vi "Angle.vi"() -> ()   [LabVIEW 2012]
panel:
  in  "Camera view angle":dbl[](array[numeric])=[48.0, 43.5]
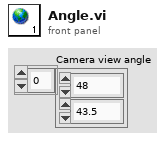
[diagram p1: front panel]
diagram:
